vi "getSpeed.vi"(8 "error in (no error)":errorcluster caption="错误输入（无错误）", 11 "OneMotion 输入":refnum<class "OneMotion.lvclass">) -> (0 "error out":errorcluster caption="错误输出", 2 "speed":i32, 3 "OneMotion 输出":refnum<class "OneMotion.lvclass">)   [LabVIEW 2016, in "MotionControl_UFO_3DOF.lvlib" / "OneMotion.lvclass"]
uses:
  <userlib>/MotionControl_UFO_3DOF/OneMotion/OneMotion.lvclass
  <userlib>/MotionControl_UFO_3DOF/OneMotion/OneMotion.lvclass/OneMotion.ctl
  <userlib>/MotionControl_UFO_3DOF/StepMotor/StepMotor.lvclass
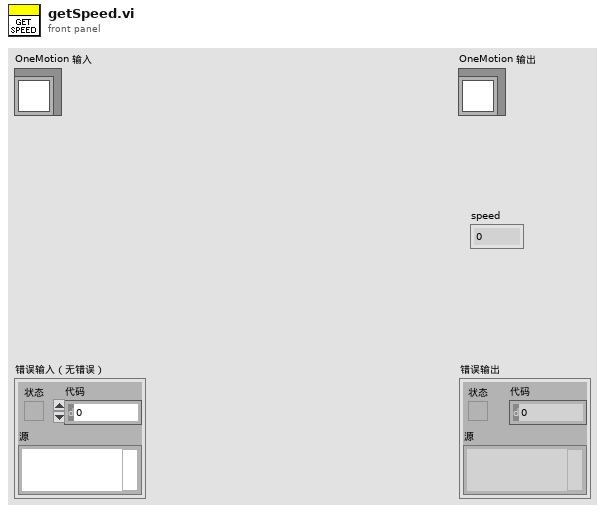
[diagram p1: front panel]
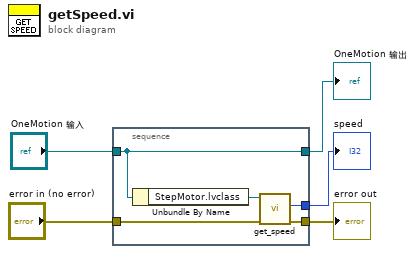
[diagram p0: block diagram]
diagram:
  n1 = stacked-sequence {
    tunnel: [w9] -> w5
    tunnel: [w6] -> w3
    tunnel: "OneMotion 输入" -> [w6]
    tunnel: [w8] -> w2
    tunnel: "error in (no error)" -> [w7]
    frame #0 {
      n2 = Unbundle By Name(w6) -> ("StepMotor.lvclass"=w10:refnum<class "StepMotor.lvclass">)
      n3 = call <userlib>:"get_speed.vi"("error in (no error)"=w7, "StepMotor 输入"=w10) -> ("error out"=w9:errorcluster, "speed"=w8:i32)  [unwired: 7 in, 1 out]
    }
  }
  "error out" <- w5
  "OneMotion 输出" <- w3
  "speed" <- w2
